vi "component_tray_region.vi"() -> ()   [LabVIEW 2021]
panel:
  out "Component Tray Region":dbl
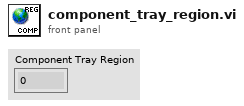
[diagram p1: front panel]
diagram:
